vi "Charger_Wake-Up All IPGs.vi"(8 "error in":errorcluster, 10 "pulse duration (3 s)":dbl[unit]=3.0, 11 "Charger COM Port":refnum<visa-resource-name>="COM17") -> (0 "error out":errorcluster)   [LabVIEW 2020]
doc: "This function enables all six charger positions twice (with a 100 ms delay between commands), sends a 3-second charge pulse, and disables all six charger positions.\n\nThe extra enable command is to improve the probability of IPG wake-up."
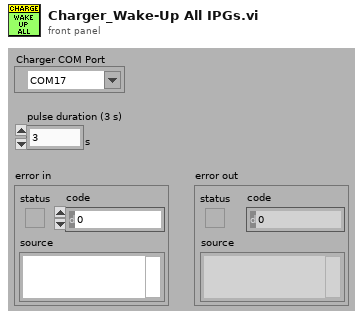
[diagram p1: front panel]
types:
  T1 = typedef "Charger_Input Control.ctl" = cluster{"address":refnum<visa-resource-name>, "position":i32, "setpoint":dbl}
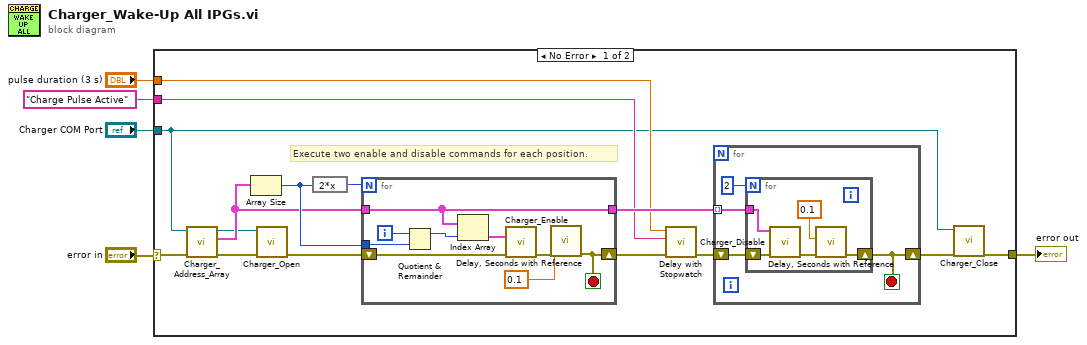
[diagram p0: block diagram]
diagram:
  n1 = case shown="No Error" "error in" {
    selector: "error in" -> [w13 w38]
    tunnel: "pulse duration (3 s)" -> [w16 _]
    tunnel: [w15 w38] -> w4
    tunnel: "Charge Pulse Active" ("window title") -> [w14 _]
    tunnel: "Charger COM Port" -> [w6 _]
    frame No Error {
      # "Execute two enable and disable commands for each position."
      n2 = call "Charger_Address_Array.vi"("error in"=w13, "Charger COM Port"=w6) -> ("error out"=w12:errorcluster, "Charger"=w8:T1[], "Charger COM dup"=w7:refnum<visa-resource-name>)  [unwired: 5 in]
      n3 = Array Size(array=w8) -> (size(s)=w9:i32)
      n4 = call "Charger_Open.vi"("error in"=w12, "Charger COM port"=w7) -> ("error out"=w11:errorcluster)  [unwired: 5 in]
      n5 = expression code="2*x"(w9) -> (w10:i32)
      n6 = for {
        N: w10 -> [_]
        shift-right: [w26] -> w19
        shift-left: w11 -> [w28]
        tunnel: w8 -> [w23]
        tunnel: [w23] -> w17
        tunnel: w9 -> [w20]
        i -> [w21]
        stop <- w26 stop-if-true
        n7 = Quotient & Remainder(x=w21, y=w20) -> (x-y*floor(x/y)=w22:i32)  [unwired: 1 out]
        n8 = Index Array(array=w23, index=w22) -> (element=w24:T1)
        n9 = call "Charger_Enable.vi"("error in"=w28, "Charger"=w24) -> ("error out"=w27:errorcluster)  [unwired: 7 in]
        n10 = call "Delay, Seconds with Reference.vi"("error in"=w27, "delay"=dbl[unit] 0.1) -> ("error out"=w26:errorcluster)  [unwired: 4 in, 2 out]
      }
      n11 = call "Delay with Stopwatch.vi"("error in"=w19, "window title"=w14, "delay"=w16) -> ("error out"=w18:errorcluster)  [unwired: 4 in]
      n12 = for {
        shift-right: [w29] -> w15
        shift-left: w18 -> [w32]
        tunnel: w17 -> [w31] mode=indexing
        stop <- w29 stop-if-true
        n13 = for {
          N: 2 -> [_]
          tunnel: w31 -> [w36]
          shift-right: [w34] -> w29
          shift-left: w32 -> [w37]
          n14 = call "Charger_Disable.vi"("error in"=w37, "Charger"=w36) -> ("error out"=w35:errorcluster)  [unwired: 7 in]
          n15 = call "Delay, Seconds with Reference.vi"("error in"=w35, "delay"=dbl[unit] 0.1) -> ("error out"=w34:errorcluster)  [unwired: 4 in, 2 out]
        }
      }
      n16 = call "Charger_Close.vi"("address"=w6) -> ()  [unwired: 6 in, 1 out]
    }
    frame Error {
    }
  }
  "error out" <- w4
